vi "Set Channel Name Waveform Attribute.vi"(8 "error in (no error)":errorcluster, 10 "DAQmx Device Name":tag, 11 "AOwfm":waveform(dbl)[](array[waveform])) -> (0 "error out":errorcluster, 3 "Array":waveform(dbl)[](array[waveform]))   [LabVIEW 2020, in "DAQmx.lvclass"]
uses:
  DAQmx.lvclass
  DAQmx.lvclass/DAQmx.ctl
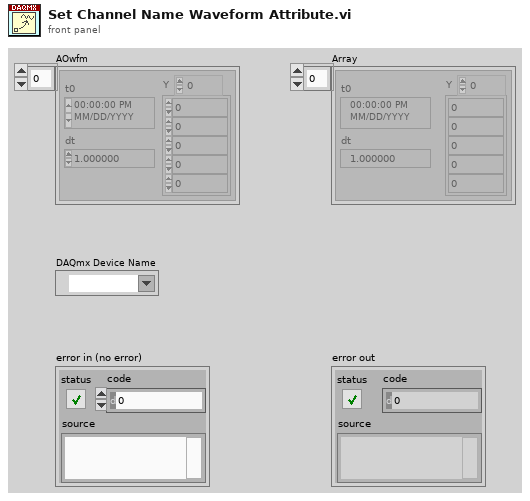
[diagram p1: front panel]
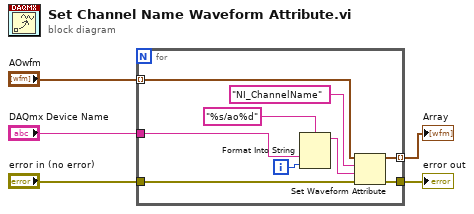
[diagram p0: block diagram]
diagram:
  n1 = for {
    tunnel: "AOwfm" -> [w13] mode=indexing
    tunnel: [w12] -> w2 mode=indexing
    tunnel: "DAQmx Device Name" -> [w8]
    tunnel: [w7] -> w4
    tunnel: "error in (no error)" -> [w6]
    i -> [w9]
    n2 = Format Into String(format string="%s/ao%d", w8, w9) -> (resulting string=w10:string)  [unwired: 2 in, 1 out]
    n3 = Set Waveform Attribute(4:w6, 5:w10, 6:"NI_ChannelName" ("name"), 7:w13) -> (0:w7:errorcluster, 3:w12:waveform(dbl))  [unwired: 1 out]
  }
  "error out" <- w4
  "Array" <- w2
